vi "Create syslog.vi"(8 "error in (no error)":errorcluster, 11 "Logger.syslog in":refnum<class "Logger.syslog.lvclass">) -> (0 "error out":errorcluster, 3 "Logger.syslog out":refnum<class "Logger.syslog.lvclass">)   [LabVIEW 2016, in "Logger.syslog.lvclass"]
uses:
  Logger.syslog.lvclass
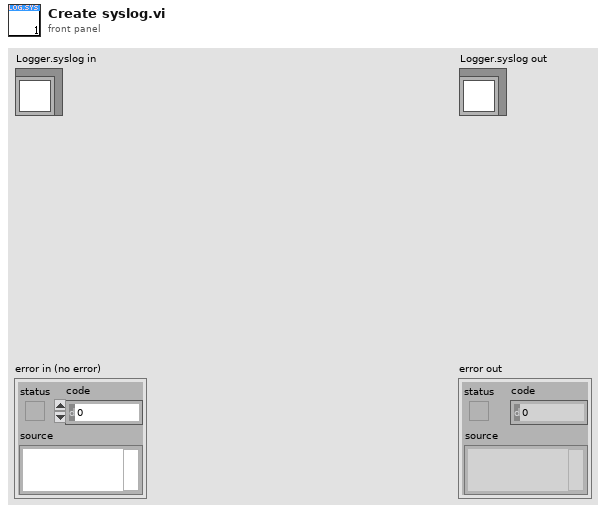
[diagram p1: front panel]
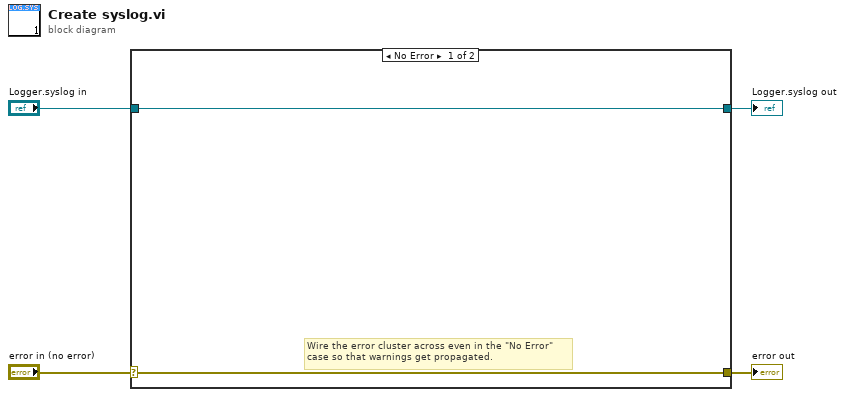
[diagram p0: block diagram]
diagram:
  n1 = case shown="No Error" "error in (no error)" {
    selector: "error in (no error)" -> [w5 w8]
    tunnel: [w5 w8] -> w3
    tunnel: [w6 w7] -> w1
    tunnel: "Logger.syslog in" -> [w6 w7]
    frame No Error {
      # "Wire the error cluster across even in the \"No Error\"\ncase so that warnings get propagated."
    }
    frame Error {
    }
  }
  "error out" <- w3
  "Logger.syslog out" <- w1
